vi "Tune.vi"(9 "Init Phase V":dbl=2.566 format="%_4g", 10 "Init Tune V":dbl=1.9 format="%_4g", 11 "Tune":bool=TRUE) -> ()   [LabVIEW 2018]
uses:
  Global 2.vi
panel:
  in  "Wideband":bool
  in  "Done":bool
  in  "Preset tune":bool
  in  "Phase Voltage":dbl=2.566 format="%_4g"
  in  "Tune Voltage":dbl=1.8849999999999991 min=0.0 max=8.0 format="%_5g"
  in  "Mode":T1(ring)
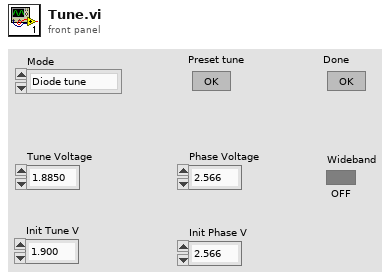
[diagram p1: front panel]
types:
  T1 = enum16{"Diode tune", "Phase tune", "Operating tune"}
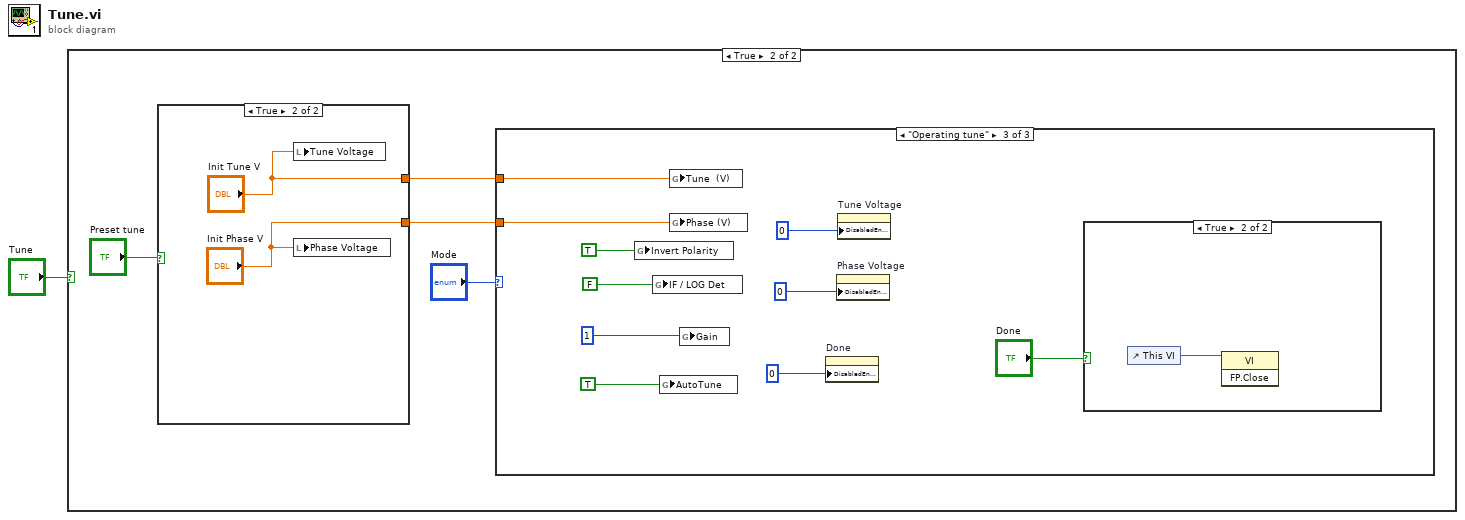
[diagram p0: block diagram]
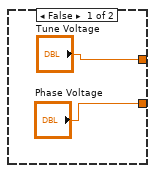
[diagram p3: hidden frame]
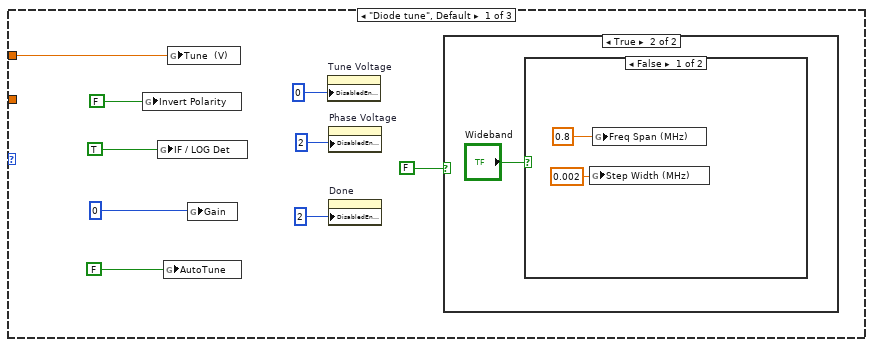
[diagram p4: hidden frame]
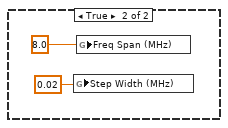
[diagram p6: hidden frame]
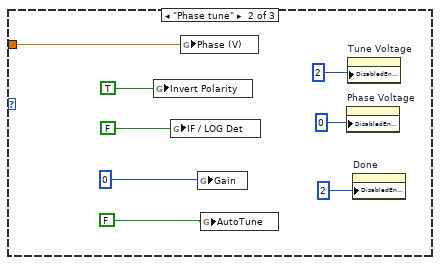
[diagram p7: hidden frame]
diagram:
  n1 = case shown="True" "Tune" {
    frame False {
    }
    frame True {
      n2 = case shown="True" "Preset tune" {
        tunnel: ["Tune Voltage" "Init Tune V"] -> w4
        tunnel: ["Phase Voltage" "Init Phase V"] -> w3
        frame False {
        }
        frame True {
          n3 = local write "Tune Voltage"("Init Tune V") -> ()
          n4 = local write "Phase Voltage"("Init Phase V") -> ()
        }
      }
      n5 = case shown="\"Operating tune\"" "Mode" {
        tunnel: w4 -> [w16 _ w41]
        tunnel: w3 -> [_ w29 w40]
        frame "Diode tune", Default {
          n6 = global write "Global 2.vi" "Invert Polarity"(FALSE) -> ()
          n7 = global write "Global 2.vi" "IF / LOG Det"(TRUE) -> ()
          n8 = global write "Global 2.vi" "AutoTune"(FALSE) -> ()
          n9 = global write "Global 2.vi" "Tune  (V)"(w16) -> ()
          n10 = global write "Global 2.vi" "Gain"(0) -> ()
          n11 = property on="Tune Voltage" class="DigNum (strict)"("DisabledEnum"=0) -> ()  [unwired: 2 in, 2 out]
          n12 = property on="Phase Voltage" class="DigNum (strict)"("DisabledEnum"=2) -> ()  [unwired: 2 in, 2 out]
          n13 = property on="Done" class="Bool (strict)"("DisabledEnum"=2) -> ()  [unwired: 2 in, 2 out]
          n14 = case shown="True" FALSE {
            frame False {
            }
            frame True {
              n15 = case shown="False" "Wideband" {
                frame False {
                  n16 = global write "Global 2.vi" "Step Width (MHz)"(0.002) -> ()
                  n17 = global write "Global 2.vi" "Freq Span (MHz)"(0.8) -> ()
                }
                frame True {
                  n18 = global write "Global 2.vi" "Step Width (MHz)"(0.02) -> ()
                  n19 = global write "Global 2.vi" "Freq Span (MHz)"(8.0) -> ()
                }
              }
            }
          }
        }
        frame "Phase tune" {
          n20 = global write "Global 2.vi" "Invert Polarity"(TRUE) -> ()
          n21 = global write "Global 2.vi" "IF / LOG Det"(FALSE) -> ()
          n22 = global write "Global 2.vi" "Phase (V)"(w29) -> ()
          n23 = global write "Global 2.vi" "Gain"(0) -> ()
          n24 = global write "Global 2.vi" "AutoTune"(FALSE) -> ()
          n25 = property on="Phase Voltage" class="DigNum (strict)"("DisabledEnum"=0) -> ()  [unwired: 2 in, 2 out]
          n26 = property on="Tune Voltage" class="DigNum (strict)"("DisabledEnum"=2) -> ()  [unwired: 2 in, 2 out]
          n27 = property on="Done" class="Bool (strict)"("DisabledEnum"=2) -> ()  [unwired: 2 in, 2 out]
        }
        frame "Operating tune" {
          n28 = global write "Global 2.vi" "Invert Polarity"(TRUE) -> ()
          n29 = global write "Global 2.vi" "IF / LOG Det"(FALSE) -> ()
          n30 = global write "Global 2.vi" "AutoTune"(TRUE) -> ()
          n31 = global write "Global 2.vi" "Tune  (V)"(w41) -> ()
          n32 = global write "Global 2.vi" "Phase (V)"(w40) -> ()
          n33 = global write "Global 2.vi" "Gain"(1) -> ()
          n34 = property on="Done" class="Bool (strict)"("DisabledEnum"=0) -> ()  [unwired: 2 in, 2 out]
          n35 = property on="Phase Voltage" class="DigNum (strict)"("DisabledEnum"=0) -> ()  [unwired: 2 in, 2 out]
          n36 = property on="Tune Voltage" class="DigNum (strict)"("DisabledEnum"=0) -> ()  [unwired: 2 in, 2 out]
          n37 = case shown="True" "Done" {
            frame False {
            }
            frame True {
              n38 = control-ref of="This VI"() -> (w42:refnum<vi>)
              n39 = invoke class="VI" method="FP.Close"(reference=w42) -> ()  [unwired: 2 in, 3 out]
            }
          }
        }
      }
    }
  }
